vi "emi_Q and Not report.vi"(11 "error in (no error)":errorcluster) -> (3 "Total in Q":i32, 8 "Sync status":T1[](array[typedef]), 14 "Error present":bool, 15 "error out":errorcluster)   [LabVIEW 2010]
uses:
  _emi_Syncronisation staus.ctl
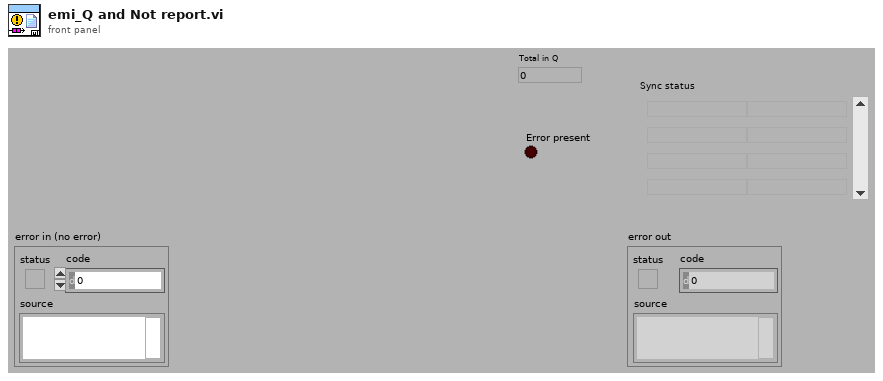
[diagram p1: front panel]
types:
  T1 = typedef "_emi_Syncronisation staus.ctl" = cluster{"Sync ID":string, "Sync Staus":string}
  T2 = enum16{"Queue", "Notifier", "Semaphore", "Rendezvous"}
  T3 = typedef "Semaphore RefNum" = refnum<k1>
  T4 = typedef "Rendezvous RefNum" = refnum<k1>
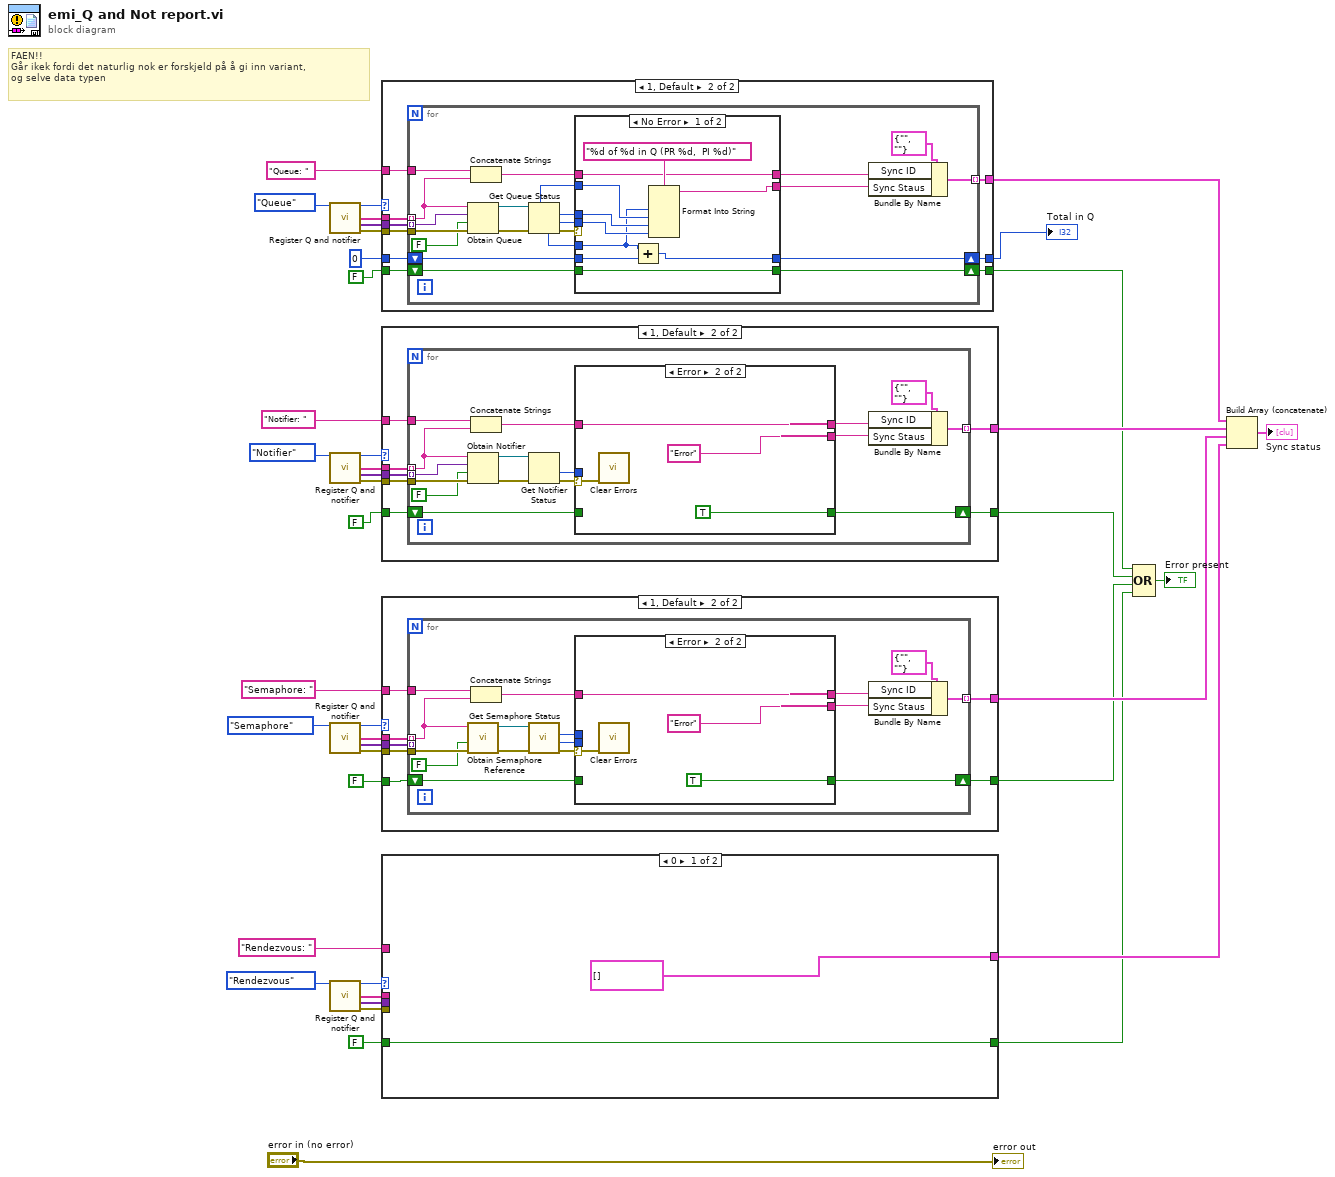
[diagram p0: block diagram]
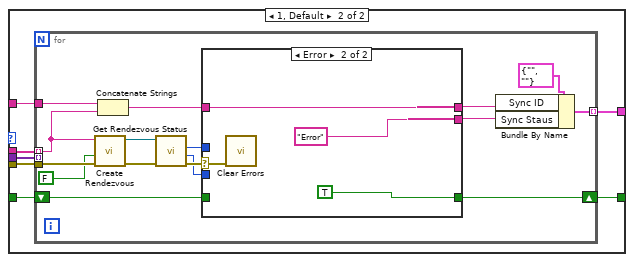
[diagram p2: hidden frame]
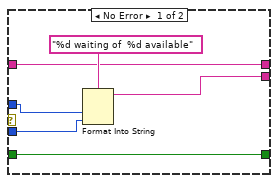
[diagram p3: hidden frame]
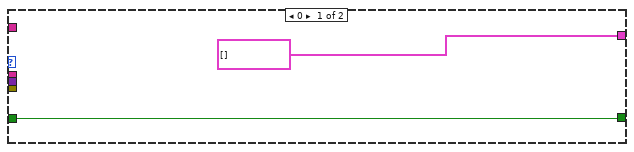
[diagram p4: hidden frame]
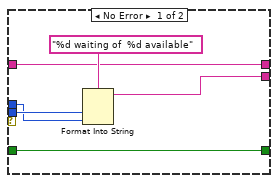
[diagram p5: hidden frame]
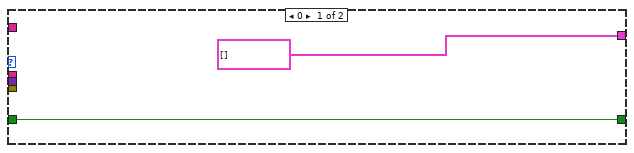
[diagram p6: hidden frame]
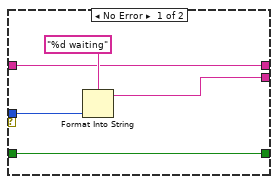
[diagram p7: hidden frame]
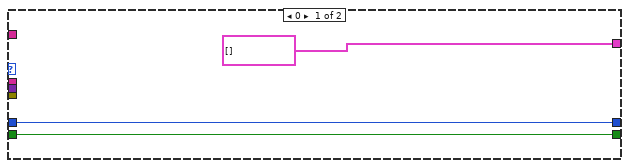
[diagram p8: hidden frame]
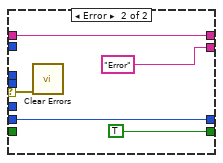
[diagram p9: hidden frame]
diagram:
  # "FAEN!!\nGår ikek fordi det naturlig nok er forskjeld på å gi inn variant,\nog selve data typen"
  n1 = call "Register Q and notifier.vi"("Type"=T2."Queue") -> ("Numb Names"=w40:i32, "Names"=w38:string[], "Types"=w37:variant[], "error out"=w39:errorcluster)  [unwired: 11 in]
  n2 = call "Register Q and notifier.vi"("Type"=T2."Notifier") -> ("Numb Names"=w33:i32, "Names"=w35:string[], "Types"=w36:variant[], "error out"=w34:errorcluster)  [unwired: 11 in]
  n3 = call "Register Q and notifier.vi"("Type"=T2."Semaphore") -> ("Numb Names"=w25:i32, "Names"=w23:string[], "Types"=w22:variant[], "error out"=w24:errorcluster)  [unwired: 11 in]
  n4 = call "Register Q and notifier.vi"("Type"=T2."Rendezvous") -> ("Numb Names"=w18:i32, "Names"=w20:string[], "Types"=w21:variant[], "error out"=w19:errorcluster)  [unwired: 11 in]
  n5 = case shown="1, Default" w40 {
    tunnel: w39 -> [_ w53]
    tunnel: w38 -> [_ w52]
    tunnel: w37 -> [_ w51]
    tunnel: "Queue: " ("Queue") -> [_ w50]
    tunnel: [T1[] [] w49] -> w29
    tunnel: 0 -> [w43 w48]
    tunnel: [w43 w47] -> w1
    tunnel: FALSE -> [w42 w46]
    tunnel: [w42 w45] -> w3
    frame 0 {
    }
    frame 1, Default {
      n6 = for {
        tunnel: w53 -> [w74]
        tunnel: w52 -> [w68] mode=indexing
        tunnel: w51 -> [w72] mode=indexing
        tunnel: w50 -> [w69]
        tunnel: [w58] -> w49 mode=indexing
        shift-right: [w56] -> w47
        shift-left: w48 -> [w57]
        shift-right: [w54] -> w45
        shift-left: w46 -> [w55]
        n7 = Obtain Queue(name (unnamed)=w68, element data type=w72, create if not found? (T)=FALSE, error in (no error)=w74) -> (queue out=w70:refnum<queue>, error out=w71:errorcluster)  [unwired: 1 in, 1 out]
        n8 = Concatenate Strings(w69, w68) -> (w66:string)
        n9 = Get Queue Status(queue=w70, error in (no error)=w71) -> (max queue size=w65:i32, # pending remove=w64:i32, # pending insert=w63:i32, error out=w67:errorcluster, # elements in queue=w62:i32)  [unwired: 1 in, 3 out]
        n10 = case shown="No Error" w67 {
          selector: w67 -> [_ w87]
          tunnel: w66 -> [w80 w89]
          tunnel: [w80 w89] -> w61
          tunnel: [w79 "Error"] -> w60
          tunnel: w65 -> [w84 _]
          tunnel: w64 -> [w83 _]
          tunnel: w63 -> [w82 _]
          tunnel: w62 -> [w77 _]
          tunnel: w57 -> [w78 w86]
          tunnel: [w76 w86] -> w56
          tunnel: w55 -> [w75 _]
          tunnel: [w75 TRUE] -> w54
          frame No Error {
            n11 = Add(x=w77, y=w78) -> (x+y=w76:i32)
            n12 = Format Into String(format string="%d of %d in Q (PR %d,  PI %d)", w77, w84, w83, w82) -> (resulting string=w79:string)  [unwired: 2 in, 1 out]
          }
          frame Error {
            n13 = call <vilib>:"Clear Errors.vi"("error in (no error)"=w87) -> ()  [unwired: 6 in, 1 out]
          }
        }
        n14 = Bundle By Name(cluster=T1 {"Sync ID"="", "Sync Staus"=""} ("output cluster"), "Sync ID"=w61, "Sync Staus"=w60) -> (w58:T1)
      }
    }
  }
  "Total in Q" <- w1
  n15 = case shown="1, Default" w33 {
    tunnel: w34 -> [_ w98]
    tunnel: w35 -> [_ w97]
    tunnel: w36 -> [_ w96]
    tunnel: [T1[] [] w94] -> w28
    tunnel: "Notifier: " ("Queue") -> [_ w95]
    tunnel: FALSE -> [w90 w93]
    tunnel: [w90 w92] -> w4
    frame 0 {
    }
    frame 1, Default {
      n16 = for {
        tunnel: w98 -> [w114]
        tunnel: w97 -> [w100] mode=indexing
        tunnel: w96 -> [w101] mode=indexing
        tunnel: w95 -> [w109]
        tunnel: [w106] -> w94 mode=indexing
        shift-right: [w103] -> w92
        shift-left: w93 -> [w102]
        n17 = Obtain Notifier(name (unnamed)=w100, notification data type=w101, create if not found? (T)=FALSE, error in (no error)=w114) -> (notifier out=w99:refnum<notifier>, error out=w112:errorcluster)  [unwired: 1 out]
        n18 = Concatenate Strings(w109, w100) -> (w108:string)
        n19 = Get Notifier Status(notifier=w99, error in (no error)=w112) -> (# waiting=w110:i32, error out=w111:errorcluster)  [unwired: 3 out]
        n20 = case shown="Error" w111 {
          selector: w111 -> [_ w121]
          tunnel: w108 -> [w118 w123]
          tunnel: [w118 w123] -> w105
          tunnel: [w117 "Error"] -> w104
          tunnel: w110 -> [w116 _]
          tunnel: [w115 TRUE] -> w103
          tunnel: w102 -> [w115 _]
          frame No Error {
            n21 = Format Into String(format string="%d waiting", w116) -> (resulting string=w117:string)  [unwired: 2 in, 1 out]
          }
          frame Error {
            n22 = call <vilib>:"Clear Errors.vi"("error in (no error)"=w121) -> ()  [unwired: 6 in, 1 out]
          }
        }
        n23 = Bundle By Name(cluster=T1 {"Sync ID"="", "Sync Staus"=""} ("output cluster"), "Sync ID"=w105, "Sync Staus"=w104) -> (w106:T1)
      }
    }
  }
  n24 = case shown="1, Default" w25 {
    tunnel: w24 -> [_ w132]
    tunnel: w23 -> [_ w131]
    tunnel: w22 -> [_ w130]
    tunnel: [T1[] [] w128] -> w15
    tunnel: "Semaphore: " ("Queue") -> [_ w129]
    tunnel: FALSE -> [w124 w127]
    tunnel: [w124 w126] -> w5
    frame 0 {
    }
    frame 1, Default {
      n25 = for {
        tunnel: w132 -> [w148]
        tunnel: w131 -> [w142] mode=indexing
        tunnel: w130 -> [_] mode=indexing
        tunnel: w129 -> [w143]
        tunnel: [w139] -> w128 mode=indexing
        shift-right: [w134] -> w126
        shift-left: w127 -> [w133]
        n26 = call <vilib>:"Obtain Semaphore Reference.vi"("error in (no error)"=w148, "create if not found (T)"=FALSE ("create if not found? (T)"), "name (unnamed)"=w142) -> ("error out"=w146:errorcluster, "semaphore"=w136:T3)  [unwired: 2 in, 1 out]
        n27 = Concatenate Strings(w143, w142) -> (w141:string)
        n28 = call <vilib>:"Get Semaphore Status.vi"("error in (no error)"=w146, "semaphore"=w136) -> ("error out"=w145:errorcluster, "# waiting"=w144:i32, "# available"=w135:i32)  [unwired: 4 in, 3 out]
        n29 = case shown="Error" w145 {
          selector: w145 -> [_ w156]
          tunnel: w141 -> [w153 w158]
          tunnel: [w153 w158] -> w138
          tunnel: [w152 "Error"] -> w137
          tunnel: w144 -> [w151 _]
          tunnel: w135 -> [w150 _]
          tunnel: [w149 TRUE] -> w134
          tunnel: w133 -> [w149 _]
          frame No Error {
            n30 = Format Into String(format string="%d waiting of  %d available", w151, w150) -> (resulting string=w152:string)  [unwired: 2 in, 1 out]
          }
          frame Error {
            n31 = call <vilib>:"Clear Errors.vi"("error in (no error)"=w156) -> ()  [unwired: 6 in, 1 out]
          }
        }
        n32 = Bundle By Name(cluster=T1 {"Sync ID"="", "Sync Staus"=""} ("output cluster"), "Sync ID"=w138, "Sync Staus"=w137) -> (w139:T1)
      }
    }
  }
  n33 = case shown="0" w18 {
    tunnel: w19 -> [_ w167]
    tunnel: w20 -> [_ w166]
    tunnel: w21 -> [_ w165]
    tunnel: [T1[] [] w163] -> w14
    tunnel: "Rendezvous: " ("Queue") -> [_ w164]
    tunnel: FALSE -> [w159 w162]
    tunnel: [w159 w161] -> w6
    frame 0 {
    }
    frame 1, Default {
      n34 = for {
        tunnel: w167 -> [w183]
        tunnel: w166 -> [w178] mode=indexing
        tunnel: w165 -> [_] mode=indexing
        tunnel: w164 -> [w179]
        tunnel: [w175] -> w163 mode=indexing
        shift-right: [w168] -> w161
        shift-left: w162 -> [w169]
        n35 = call <vilib>:"Create Rendezvous.vi"("error in (no error)"=w183, "return existing (F)"=FALSE ("create if not found? (T)"), "name (unnamed)"=w178) -> ("error out"=w181:errorcluster, "rendezvous"=w172:T4)  [unwired: 2 in, 1 out]
        n36 = Concatenate Strings(w179, w178) -> (w177:string)
        n37 = call <vilib>:"Get Rendezvous Status.vi"("error in (no error)"=w181, "rendezvous"=w172) -> ("error out"=w180:errorcluster, "size"=w170:i32, "# waiting"=w171:i32)  [unwired: 5 in, 2 out]
        n38 = case shown="Error" w180 {
          selector: w180 -> [_ w191]
          tunnel: w177 -> [w188 w193]
          tunnel: [w188 w193] -> w174
          tunnel: [w187 "Error"] -> w173
          tunnel: w171 -> [w186 _]
          tunnel: w170 -> [w185 _]
          tunnel: w169 -> [w184 _]
          tunnel: [w184 TRUE] -> w168
          frame No Error {
            n39 = Format Into String(format string="%d waiting of  %d available", w186, w185) -> (resulting string=w187:string)  [unwired: 2 in, 1 out]
          }
          frame Error {
            n40 = call <vilib>:"Clear Errors.vi"("error in (no error)"=w191) -> ()  [unwired: 6 in, 1 out]
          }
        }
        n41 = Bundle By Name(cluster=T1 {"Sync ID"="", "Sync Staus"=""} ("output cluster"), "Sync ID"=w174, "Sync Staus"=w173) -> (w175:T1)
      }
    }
  }
  n42 = Compound Arithmetic op=OR(w3, w4, w5, w6) -> (→"Error present":bool)
  n43 = Build Array (concatenate)(w29, w28, w15, w14) -> (→"Sync status":T1[])
  "error out" <- "error in (no error)"
